vi "Untitled 1 (SubVI).vi"(11 "Ultrasonic 01":dbl) -> (3 "Numeric":dbl)   [LabVIEW 2020]
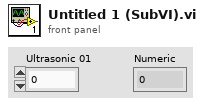
[diagram p1: front panel]
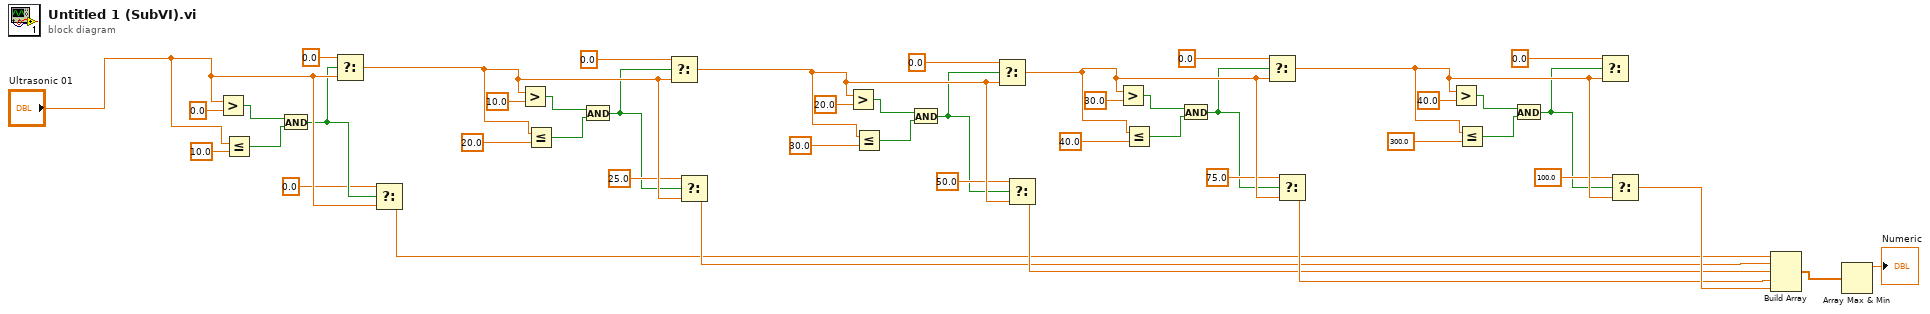
[diagram p0: block diagram]
diagram:
  n1 = Greater?(x="Ultrasonic 01", y=0.0) -> (0:w3:bool)
  n2 = Less Or Equal?(x="Ultrasonic 01", y=10.0) -> (x <= y?=w4:bool)
  n3 = And(x=w3, y=w4) -> (x .and. y?=w11:bool)
  n4 = Select(t=0.0, s=w11, f="Ultrasonic 01") -> (s? t:f=w15:dbl)
  n5 = Select(t=0.0, s=w11, f="Ultrasonic 01") -> (s? t:f=w41:dbl)
  n6 = Greater?(x=w15, y=10.0) -> (0:w7:bool)
  n7 = Less Or Equal?(x=w15, y=20.0) -> (x <= y?=w8:bool)
  n8 = And(x=w7, y=w8) -> (x .and. y?=w13:bool)
  n9 = Select(t=0.0, s=w13, f=w15) -> (s? t:f=w23:dbl)
  n10 = Select(t=25.0, s=w13, f=w15) -> (s? t:f=w42:dbl)
  n11 = Greater?(x=w23, y=20.0) -> (0:w18:bool)
  n12 = Less Or Equal?(x=w23, y=30.0) -> (x <= y?=w19:bool)
  n13 = And(x=w18, y=w19) -> (x .and. y?=w21:bool)
  n14 = Select(t=0.0, s=w21, f=w23) -> (s? t:f=w31:dbl)
  n15 = Select(t=50.0, s=w21, f=w23) -> (s? t:f=w43:dbl)
  n16 = Greater?(x=w31, y=30.0) -> (0:w26:bool)
  n17 = Less Or Equal?(x=w31, y=40.0) -> (x <= y?=w27:bool)
  n18 = And(x=w26, y=w27) -> (x .and. y?=w29:bool)
  n19 = Select(t=0.0, s=w29, f=w31) -> (s? t:f=w39:dbl)
  n20 = Select(t=75.0, s=w29, f=w31) -> (s? t:f=w44:dbl)
  n21 = Greater?(x=w39, y=40.0) -> (0:w34:bool)
  n22 = Less Or Equal?(x=w39, y=300.0) -> (x <= y?=w35:bool)
  n23 = And(x=w34, y=w35) -> (x .and. y?=w37:bool)
  n24 = Select(t=0.0, s=w37, f=w39) -> ()  [unwired: 1 out]
  n25 = Select(t=100.0, s=w37, f=w39) -> (s? t:f=w45:dbl)
  n26 = Build Array(w41, w42, w43, w44, w45) -> (w46:dbl[])
  n27 = Array Max & Min(array=w46) -> (max value=→"Numeric":dbl)  [unwired: 3 out]
